vi "Clear.vi"(8 "error in (no error)":errorcluster) -> (0 "error out":errorcluster)   [LabVIEW 2015, in "ReplayBot.lvlib"]
uses:
  ReplayBot.lvlib
  ReplayQueueFGV_Command.ctl
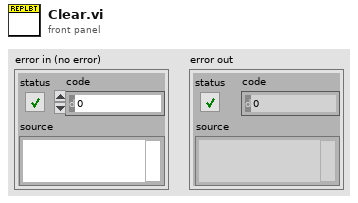
[diagram p1: front panel]
types:
  T1 = typedef "ReplayBot.lvlib/ReplayQueueFGV_Command.ctl" = enum16{"ObtainQueue", "ReleaseAllQueues"}
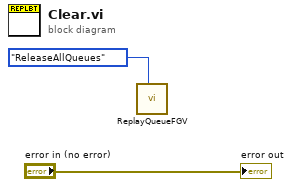
[diagram p0: block diagram]
diagram:
  n1 = call "ReplayQueueFGV.vi"("Command (ObtainQueue)"=ReplayQueueFGV_Command."ReleaseAllQueues") -> ()  [unwired: 10 in, 1 out]
  "error out" <- "error in (no error)"
